vi "ChangeGrating.vi"(8 "error in (no error)":errorcluster, 10 "Grating":enum16{"Mirror", "1200 g/mm", "1800 g/mm"}(ring), 11 "HRS_Spectrometer in":refnum<class "HRS_Spectrometer.lvclass">) -> (0 "error out":errorcluster, 3 "HRS_Spectrometer out":refnum<class "HRS_Spectrometer.lvclass">)   [LabVIEW 2023, in "HRS_Spectrometer.lvlib" / "HRS_Spectrometer.lvclass"]
uses:
  HRS_Spectrometer.lvclass
  HRS_Spectrometer.lvclass/HRS_Spectrometer.ctl
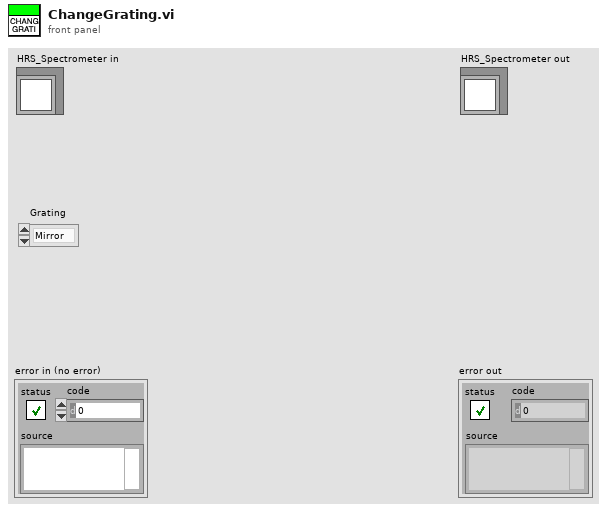
[diagram p1: front panel]
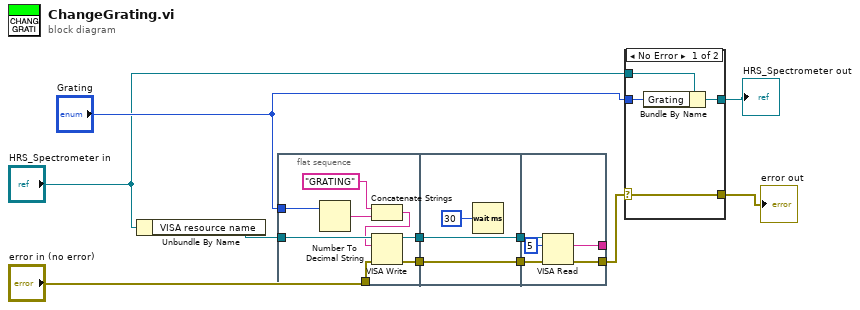
[diagram p0: block diagram]
diagram:
  n1 = Unbundle By Name("HRS_Spectrometer in") -> ("VISA resource name"=w4:refnum<visa-resource-name>)
  n2 = flat-sequence {
    tunnel: [w19] -> w11
    tunnel: [w18] -> w10
    tunnel: "Grating" -> [w15]
    tunnel: w4 -> [w14]
    tunnel: "error in (no error)" -> [w13]
    tunnel: w11 -> [w22]
    tunnel: w10 -> [w21]
    tunnel: [w22] -> w9
    tunnel: [w21] -> w8
    tunnel: w9 -> [w26]
    tunnel: w8 -> [w27]
    tunnel: [w25] -> _
    tunnel: [w24] -> w7
    frame #0 {
      n3 = Number To Decimal String(number=w15) -> (decimal integer string=w16:string)  [unwired: 1 in]
      n4 = Concatenate Strings("GRATING" ("write buffer"), w16) -> (w12:string)
      n5 = VISA Write(VISA resource name=w14, write buffer=w12, error in (no error)=w13) -> (VISA resource name out=w19:refnum<visa-resource-name>, error out=w18:errorcluster)  [unwired: 1 out]
    }
    frame #1 {
      n6 = Wait (ms)(milliseconds to wait=u32 30) -> ()  [unwired: 1 out]
    }
    frame #2 {
      n7 = VISA Read(VISA resource name=w26, byte count=u32 5, error in (no error)=w27) -> (read buffer=w25:string, error out=w24:errorcluster)  [unwired: 2 out]
    }
  }
  n8 = case shown="No Error" w7 {
    selector: w7 -> [w28 w32]
    tunnel: "HRS_Spectrometer in" -> [w31 w33]
    tunnel: "Grating" -> [w30 _]
    tunnel: [w29 w33] -> w5
    tunnel: [w28 w32] -> w1
    frame No Error {
      n9 = Bundle By Name(cluster=w31, "Grating"=w30) -> (w29:refnum<class "HRS_Spectrometer.lvclass">)
    }
    frame Error {
    }
  }
  "error out" <- w1
  "HRS_Spectrometer out" <- w5
